vi "get segment count out from waveform.vi"() -> ()   [LabVIEW 2013]
panel:
  out "0 to 4 particle count 2":T1
  in  "count bottom":i32[](graph)
  in  "count top":i32[](graph)
  out "0 to 4 particle count":T1
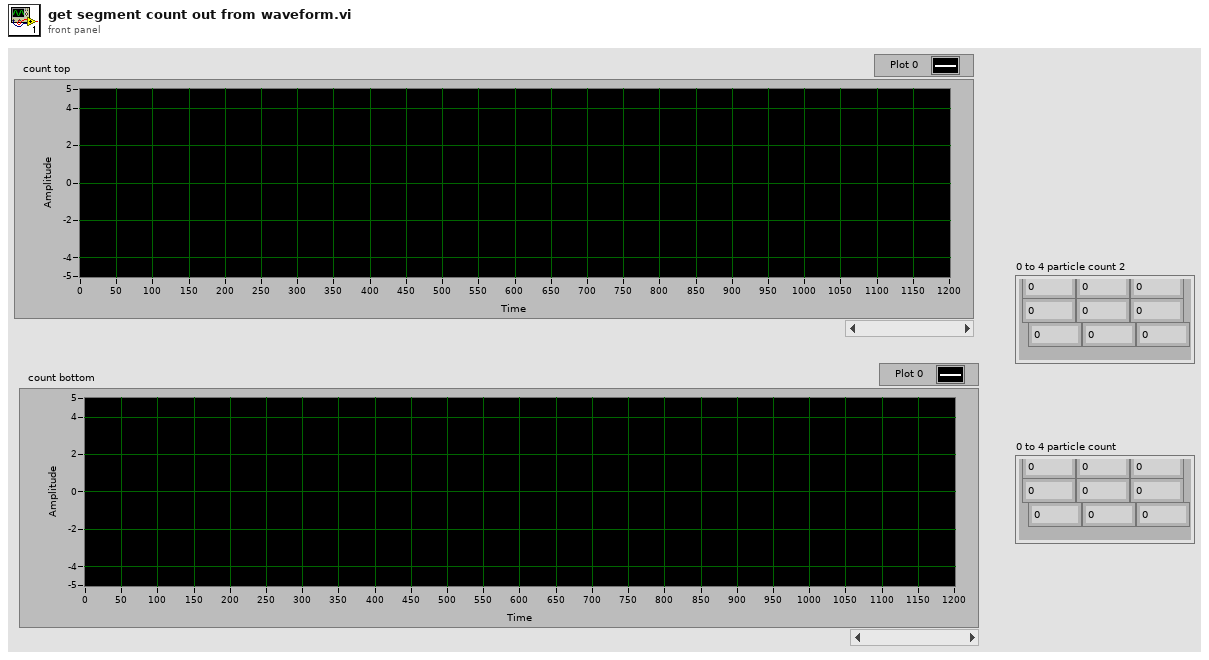
[diagram p1: front panel]
types:
  T1 = cluster{i32, i32, i32, i32, i32, i32, i32, i32, i32}
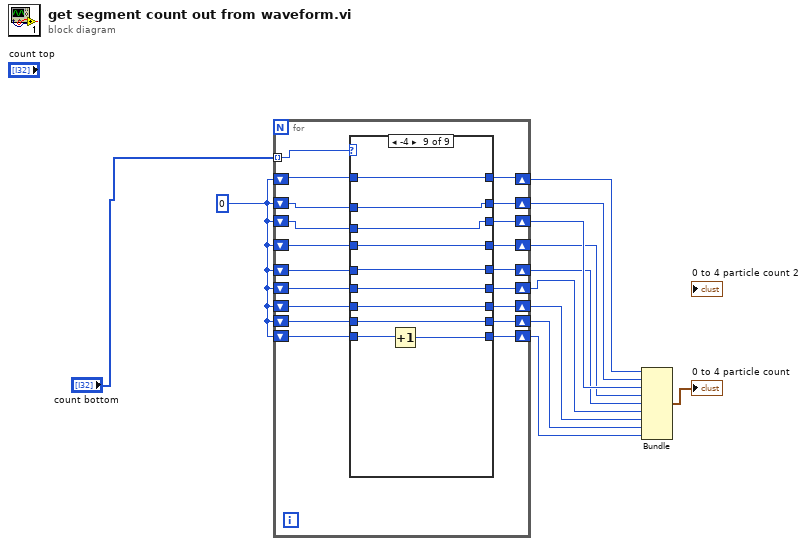
[diagram p0: block diagram]
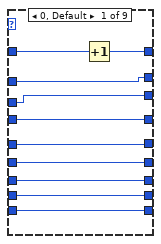
[diagram p2: hidden frame]
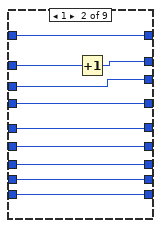
[diagram p3: hidden frame]
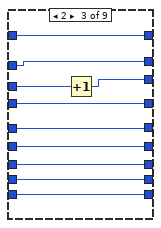
[diagram p4: hidden frame]
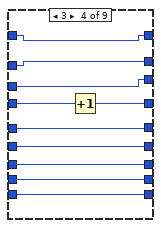
[diagram p5: hidden frame]
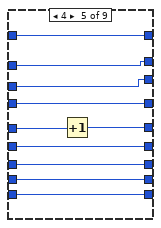
[diagram p6: hidden frame]
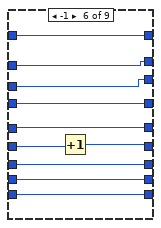
[diagram p7: hidden frame]
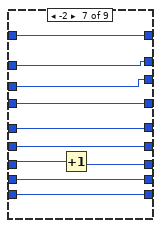
[diagram p8: hidden frame]
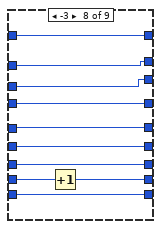
[diagram p9: hidden frame]
diagram:
  w7 = 0
  n1 = for {
    tunnel: "count bottom" -> [w31] mode=indexing
    shift-right: [w27] -> w11
    shift-left: w7 -> [w28]
    shift-right: [w30] -> w12
    shift-left: w7 -> [w29]
    shift-right: [w25] -> w10
    shift-left: w7 -> [w26]
    shift-right: [w23] -> w9
    shift-left: w7 -> [w24]
    shift-right: [w21] -> w8
    shift-left: w7 -> [w22]
    shift-right: [w16] -> w6
    shift-left: w7 -> [w20]
    shift-right: [w15] -> w5
    shift-left: w7 -> [w19]
    shift-right: [w14] -> w4
    shift-left: w7 -> [w18]
    shift-right: [w13] -> w3
    shift-left: w7 -> [w17]
    n2 = case shown="-4" w31 {
      tunnel: [w41 w49 w59 w69 w79 w91 w101 w111 w121] -> w30
      tunnel: w29 -> [w40 w49 w59 w69 w79 w91 w101 w111 w121]
      tunnel: w28 -> [w39 w51 w58 w68 w78 w90 w100 w110 w120]
      tunnel: [w39 w50 w58 w68 w78 w90 w100 w110 w120] -> w27
      tunnel: w26 -> [w38 w48 w61 w67 w77 w89 w99 w109 w119]
      tunnel: [w38 w48 w60 w67 w77 w89 w99 w109 w119] -> w25
      tunnel: w24 -> [w37 w47 w57 w71 w76 w88 w98 w108 w118]
      tunnel: [w37 w47 w57 w70 w76 w88 w98 w108 w118] -> w23
      tunnel: w22 -> [w36 w46 w56 w66 w81 w84 w94 w102 w112]
      tunnel: [w36 w46 w56 w66 w80 w84 w94 w102 w112] -> w21
      tunnel: w20 -> [w35 w45 w55 w65 w75 w83 w97 w107 w117]
      tunnel: w19 -> [w34 w44 w54 w64 w74 w87 w92 w106 w116]
      tunnel: w18 -> [w33 w43 w53 w63 w73 w86 w96 w104 w115]
      tunnel: w17 -> [w32 w42 w52 w62 w72 w85 w95 w105 w114]
      tunnel: [w35 w45 w55 w65 w75 w82 w97 w107 w117] -> w16
      tunnel: [w34 w44 w54 w64 w74 w87 w93 w106 w116] -> w15
      tunnel: [w33 w43 w53 w63 w73 w86 w96 w103 w115] -> w14
      tunnel: [w32 w42 w52 w62 w72 w85 w95 w105 w113] -> w13
      frame 0, Default {
        n3 = Increment(x=w40) -> (x+1=w41:i32)
      }
      frame 1 {
        n4 = Increment(x=w51) -> (x+1=w50:i32)
      }
      frame 2 {
        n5 = Increment(x=w61) -> (x+1=w60:i32)
      }
      frame 3 {
        n6 = Increment(x=w71) -> (x+1=w70:i32)
      }
      frame 4 {
        n7 = Increment(x=w81) -> (x+1=w80:i32)
      }
      frame -1 {
        n8 = Increment(x=w83) -> (x+1=w82:i32)
      }
      frame -2 {
        n9 = Increment(x=w92) -> (x+1=w93:i32)
      }
      frame -3 {
        n10 = Increment(x=w104) -> (x+1=w103:i32)
      }
      frame -4 {
        n11 = Increment(x=w114) -> (x+1=w113:i32)
      }
    }
  }
  n12 = Bundle(w12, w11, w10, w9, w8, w6, w5, w4, w3) -> (→"0 to 4 particle count":T1)  [unwired: 1 in]
